vi "Pixel Map.vi"(8 "error in":errorcluster, 10 "Pixel Map":bool, 11 "ImageHandler in":refnum<class "ImageHandler.lvclass">) -> (0 "error out":errorcluster, 3 "ImageHandler out":refnum<class "ImageHandler.lvclass">)   [LabVIEW 2022 SP3, in "ImageHandler.lvlib" / "ImageHandler.lvclass"]
uses:
  ImageHandler.lvclass
  ImageHandler.lvclass/ImageHandler.ctl
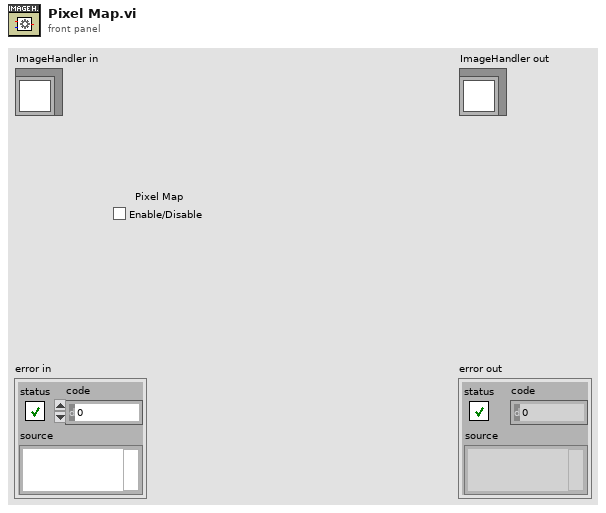
[diagram p1: front panel]
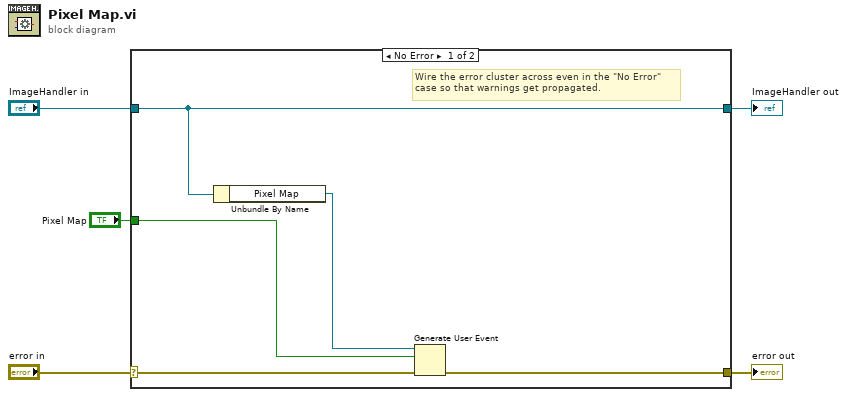
[diagram p0: block diagram]
diagram:
  n1 = case shown="No Error" "error in" {
    selector: "error in" -> [w10 w12]
    tunnel: [w9 w12] -> w4
    tunnel: [w8 w11] -> w2
    tunnel: "ImageHandler in" -> [w8 w11]
    tunnel: "Pixel Map" -> [w6 _]
    frame No Error {
      # "Wire the error cluster across even in the \"No Error\"\ncase so that warnings get propagated."
      n2 = Unbundle By Name(w8) -> ("Pixel Map"=w7:refnum<user-event>)
      n3 = Generate User Event(user event=w7, event data cluster=w6, error in=w10) -> (error out=w9:errorcluster)  [unwired: 1 in, 1 out]
    }
    frame Error {
    }
  }
  "error out" <- w4
  "ImageHandler out" <- w2
